vi "Deserialize Waypoint Array.vi"(11 "Serialized Waypoint Array":string) -> (2 "Waypoints Object Array":T1, 3 "Waypoints Array":T2[](array[typedef]) {"UTM Location"."North" format="%#_10f"; "UTM Location"."East" format="%#_8f"})   [LabVIEW 2011, in "Waypoint.lvclass"]
uses:
  Waypoint.lvclass
  0x2-OCU-Think Comm/0x2 Typedefs/ocuWaypoint.ctl
  2 Typedefs/UTM Location.ctl
  0x2-OCU-Think Comm/0x2 Typedefs/Waypoints List.ctl
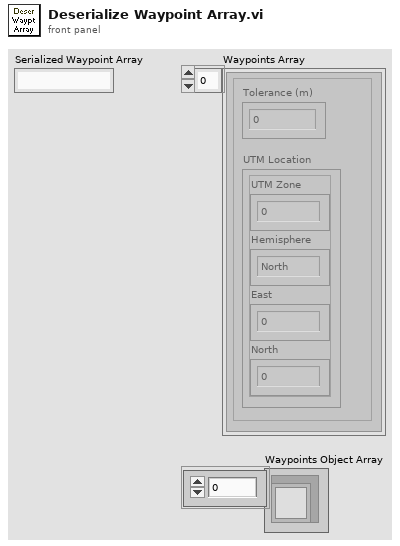
[diagram p1: front panel]
types:
  T1 = typedef "Waypoints List.ctl" = refnum<class "Waypoint.lvclass">[]
  T2 = typedef "ocuWaypoint.ctl" = cluster{"Tolerance (m)":dbl, "UTM Location":T3}
  T3 = typedef "UTM Location.ctl" = cluster{"UTM Zone":dbl, "Hemisphere":enum16{"North", "South"}, "East":dbl, "North":dbl}
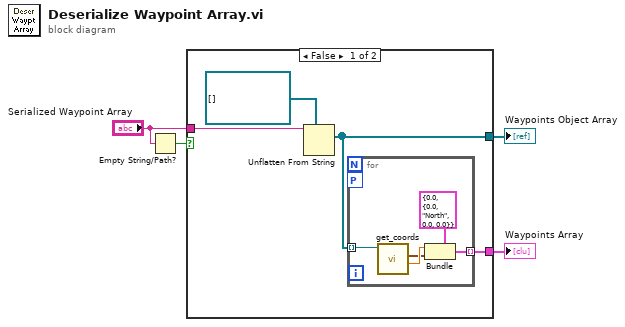
[diagram p0: block diagram]
diagram:
  n1 = Empty String/Path?(string/path="Serialized Waypoint Array") -> (empty?=w1:bool)
  n2 = case shown="False" w1 {
    tunnel: [w8 _] -> w4
    tunnel: [w7 _] -> w3
    tunnel: "Serialized Waypoint Array" -> [w5 _]
    frame False {
      n3 = Unflatten From String(type=T1 [] ("Waypoints Array"), binary string=w5) -> (value=w7:T1)  [unwired: 3 in, 2 out]
      n4 = for {
        tunnel: w7 -> [w13] mode=indexing
        workers-P: _ -> [_]
        tunnel: [w9] -> w8 mode=indexing
        n5 = call-dynamic "get_coords.vi"("Waypoint in"=w13) -> ("Tolerance (meters?)"=w12:dbl, "Coords"=w11:T3)  [unwired: 7 in, 2 out]
        n6 = Bundle(cluster=T2 {"Tolerance (m)"=0.0, "UTM Location"={"UTM Zone"=0.0, "Hemisphere"=enum."North", "East"=0.0, "North"=0.0}} ("Waypoint"), "Tolerance (m)"=w12, "UTM Location"=w11) -> (w9:T2)
      }
    }
    frame True {
    }
  }
  "Waypoints Array" <- w4
  "Waypoints Object Array" <- w3
